vi "ASI_Quit.vi"(11 "VISA Refnum in":refnum<visa-resource-name>) -> ()   [LabVIEW 2011]
panel:
  out "read buffer":string
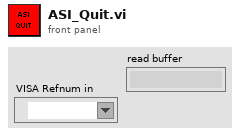
[diagram p1: front panel]
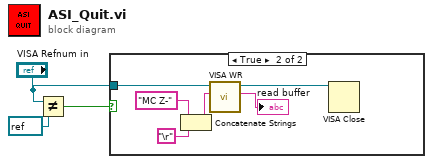
[diagram p0: block diagram]
diagram:
  n1 = Not Equal?(x="VISA Refnum in", y=refnum<visa-resource-name> refnum ("VISA resource name")) -> (x != y?=w1:bool)
  n2 = case shown="True" w1 {
    tunnel: "VISA Refnum in" -> [_ w9]
    frame False {
    }
    frame True {
      n3 = Concatenate Strings("MC Z-" ("write buffer"), "\r") -> (w6:string)
      n4 = call "VISA WR.vi"("write buffer"=w6, "VISA Refnum in"=w9) -> ("read buffer"=→"read buffer":string, "VISA Refnum out"=w8:refnum<visa-resource-name>)  [unwired: 7 in, 1 out]
      n5 = VISA Close(VISA resource name=w8) -> ()  [unwired: 1 in, 1 out]
    }
  }
